vi "Analysis Dialog.vi"(8 "error in (no error)":errorcluster, 10 "Test Results":T5, 11 "Database in":refnum<queue>) -> (0 "error IO":errorcluster, 3 "Database out":refnum<queue>)   [LabVIEW 2026, in "Analysis.lvlib"]
uses:
  Analysis.lvlib
  Test Results.ctl
  Test Details.ctl
  support/Architecture/Message Queue/Message Cluster.ctl
  Hysteresis Result.ctl
  Repeatability Result.ctl
  Accuracy Result.ctl
  Linearity Result.ctl
  controls/UI/Analytics Refs.ctl
  controls/UI/UI List Type.ctl
  <vilib>/Utility/NIReport.llb/Report Type.ctl
  <vilib>/Utility/NIReport.llb/Append Text Table to Report (wrap).vi
  <vilib>/printing/OpenHTMLReport.llb/Open HTML Report in Browser (Refnum).vi
  <vilib>/Utility/NIReport.llb/NI_report.lvclass
  Settings/Settings.lvlib
  <vilib>/Utility/NIReport.llb/NI_ReportGenerationCore.lvlib
  support/Architecture/Message Queue/Message Queue.lvlib
panel:
  out "Temporary HTML file created":path
  in  "Generate Report":bool
  out "Max Deviations":dbl[](array[numeric])
  out "Linearity Results":T1[](array[typedef])
  out "Accuracy Results":T2[](array[typedef])
  out "Maximum Absolute Error":dbl
  out "Max Repeatability":dbl
  out "Repeatability Results":T3[](array[typedef])
  out "Max Hysteresis":dbl
  out "Hysteresis Results":T4[](array[typedef])
  in  "Exit":bool
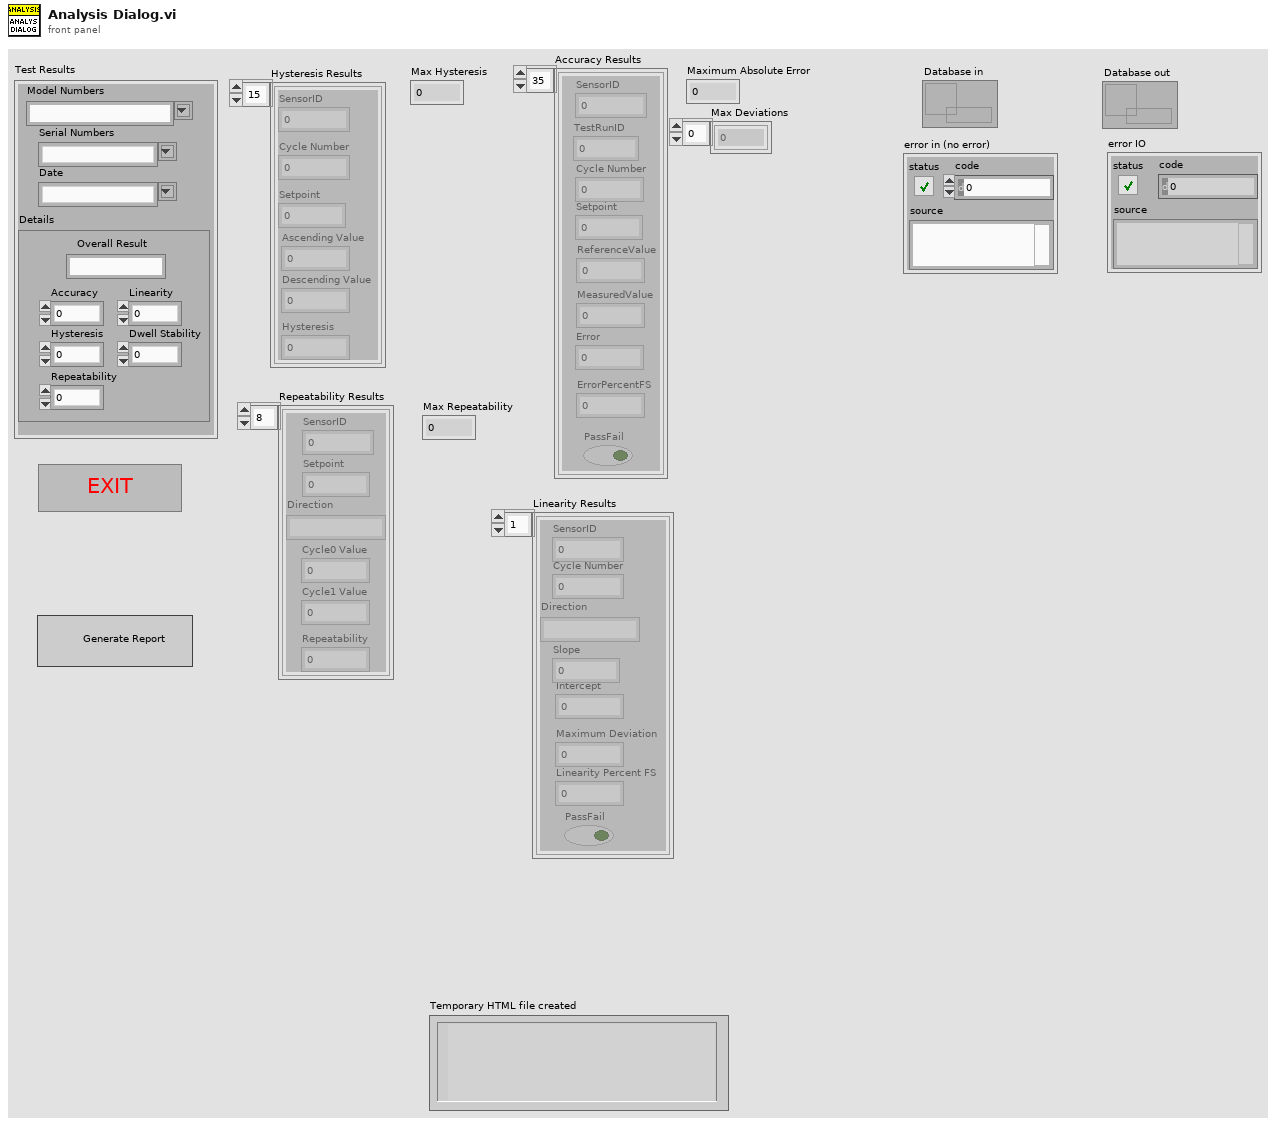
[diagram p1: front panel]
types:
  T1 = typedef "Analysis.lvlib/Linearity Result.ctl" = cluster{"Slope":dbl, "Intercept":dbl, "Cycle Number":i32, "SensorID":i32, "Maximum Deviation":dbl, "Linearity Percent FS":dbl, "Direction":string, "PassFail":bool}
  T2 = typedef "Analysis.lvlib/Accuracy Result.ctl" = cluster{"Setpoint":dbl, "Cycle Number":i32, "SensorID":i32, "TestRunID":i32, "ReferenceValue":dbl, "MeasuredValue":dbl, "ErrorPercentFS":dbl, "PassFail":bool, "Error":dbl}
  T3 = typedef "Analysis.lvlib/Repeatability Result.ctl" = cluster{"Setpoint":dbl, "Cycle0 Value":dbl, "SensorID":i32, "Cycle1 Value":dbl, "Repeatability":dbl, "Direction":string}
  T4 = typedef "Analysis.lvlib/Hysteresis Result.ctl" = cluster{"Setpoint":dbl, "Ascending Value":dbl, "Cycle Number":i32, "SensorID":i32, "Descending Value":dbl, "Hysteresis":dbl}
  T5 = typedef "Analysis.lvlib/Test Results.ctl" = cluster{"Model Numbers":string, "Serial Numbers":string, "Date":string, "Details":T6}
  T6 = typedef "Analysis.lvlib/Test Details.ctl" = cluster{"Accuracy":dbl, "Hysteresis":dbl, "Repeatability":dbl, "Linearity":dbl, "Dwell Stability":dbl, "Overall Result":string}
  T7 = typedef "Analysis.lvlib/Analytics Refs.ctl" = cluster{"Model Numbers Ref":refnum<vi>, "Serial Numbers Ref":refnum<vi>, "Date Ref":refnum<vi>, "Generate Report Ref":refnum<vi>}
  T8 = enum8{"Enabled", "Disabled", "Disabled and Grayed Out"}
  T9 = typedef "UI List Type.ctl" = enum16{"Model Numbers", "Serial Numbers", "Operators", "Calibration Points", "Start Run Times"}
  T10 = typedef "NI_ReportGenerationCore.lvlib/Report Type.ctl" = enum16{"HTML", "Word", "Excel"}
  T11 = typedef "Calibration Point Table Insert.ctl" = cluster{"TestRunID":i32, "ChannelRecordID":i32, "Setpoint":dbl, "MeasuredValue":dbl, "ErrorPercent":dbl, "PassFail":bool, "ReferenceValue":dbl, "Cycle Number":i32, "Direction":string, "SensorID":i32}
  T12 = typedef "Settings.lvlib/Sensor CoreData Cluster.ctl" = cluster{"SensorID":i32, "SerialNumber":string, "ModelNumber":string, "Min":dbl, "Max":dbl, "Units":T13, "Output Signal":T14}
  T13 = typedef "Units Enum.ctl" = enum16{"PSI", "Deg C", "kPa", "GPM"}
  T14 = typedef "Signal Enum.ctl" = enum16{"4-20mA", "0-10V", "Thermocouple Type K"}
  T15 = typedef "Analysis.lvlib/Full Scale Sensor Cluster.ctl" = cluster{"SensorID":i32, "FS":dbl}
  T16 = cluster{"Direction":string, "Cycle Number":i32, "SensorID":i32}[]
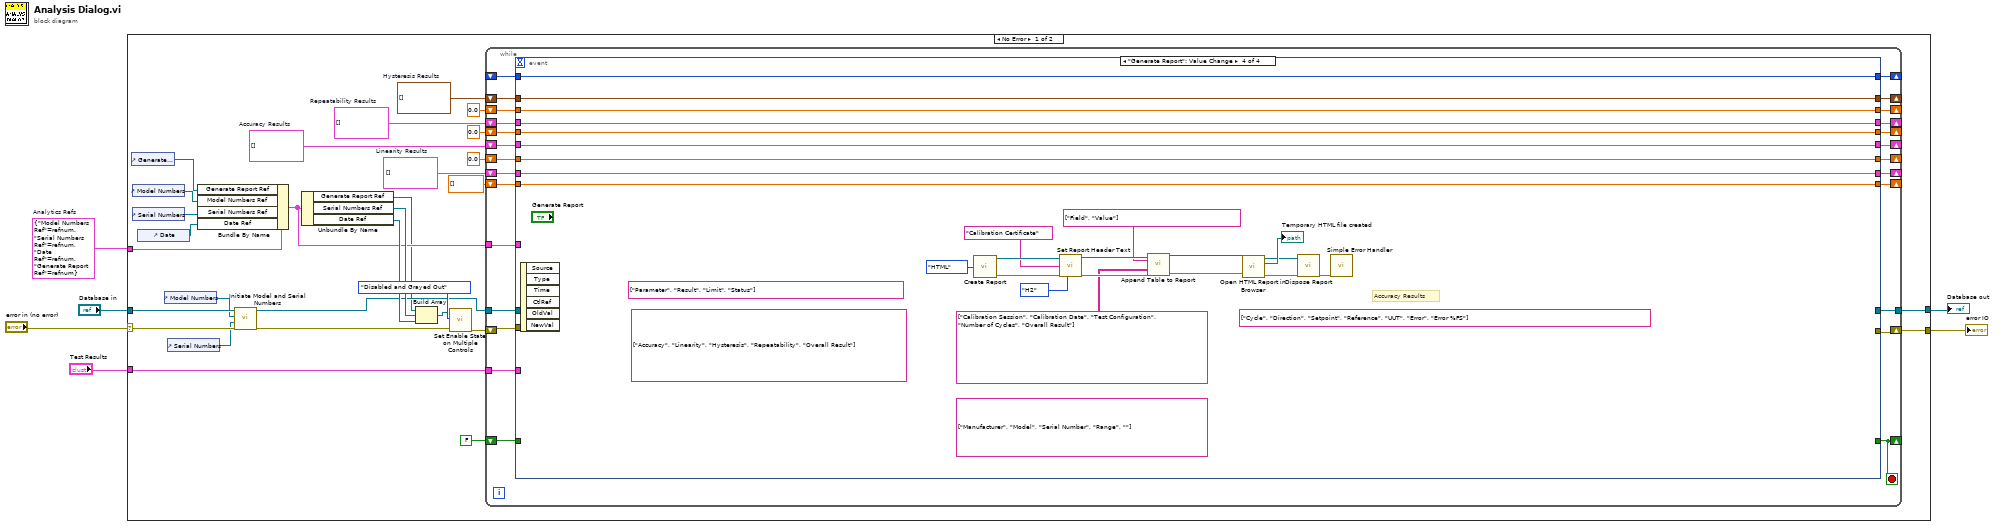
[diagram p0: block diagram]
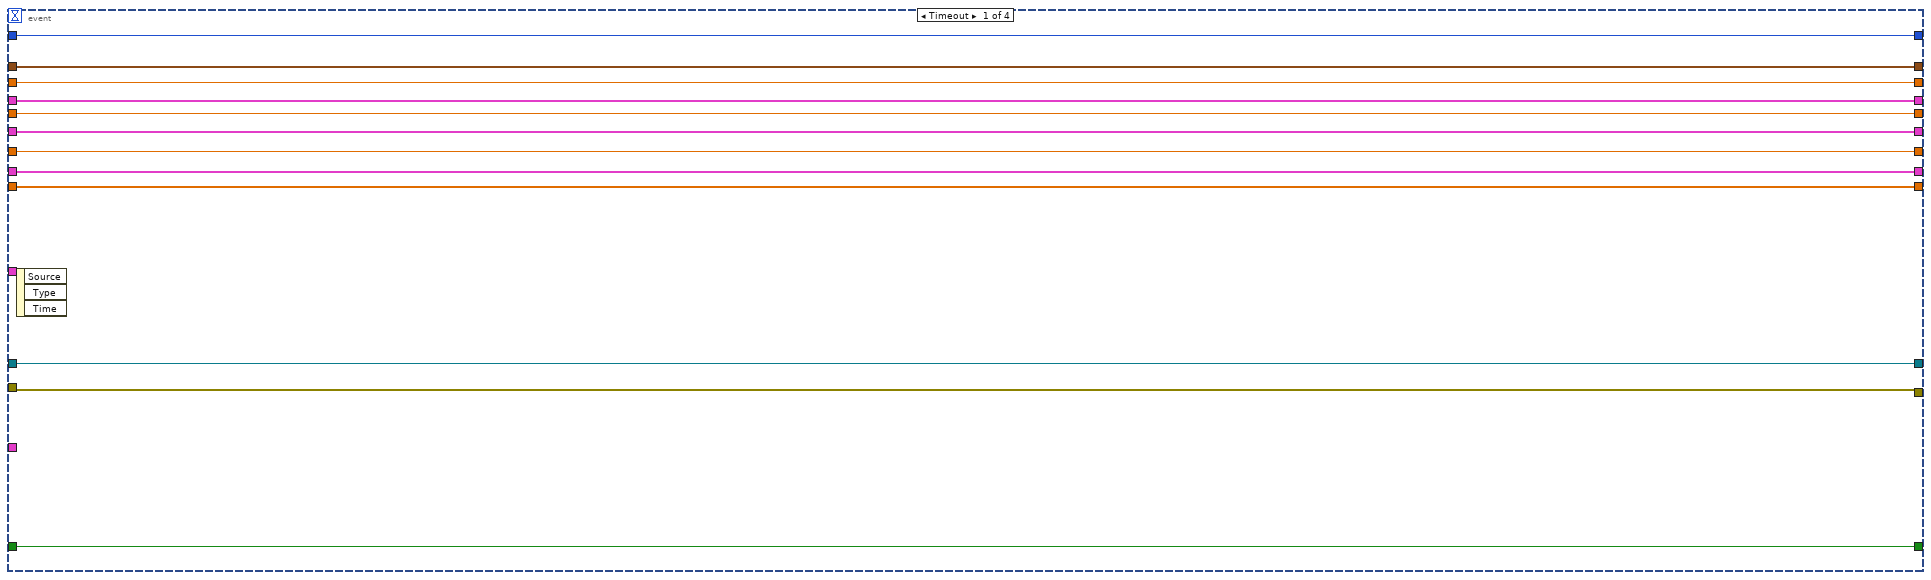
[diagram p2: hidden frame]
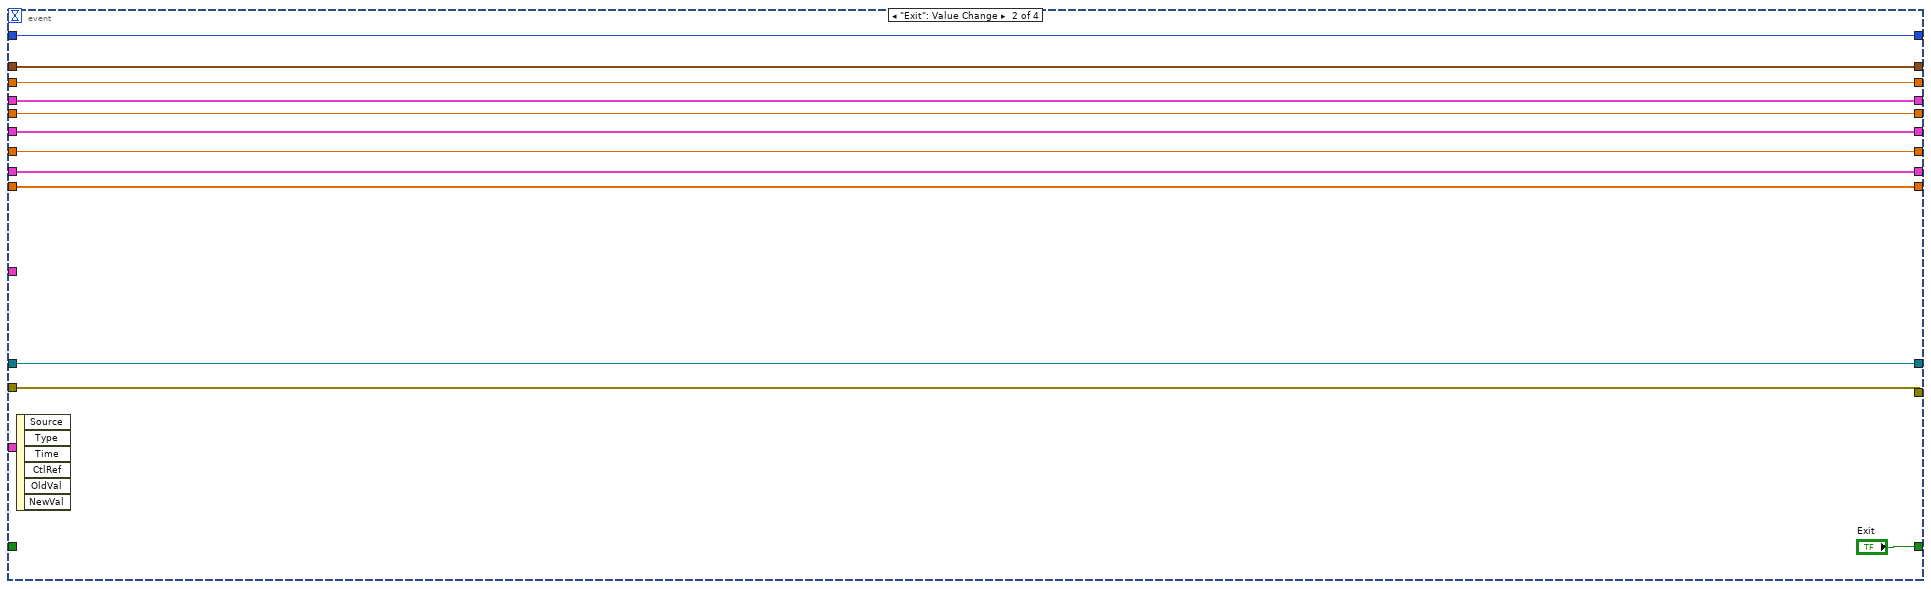
[diagram p3: hidden frame]
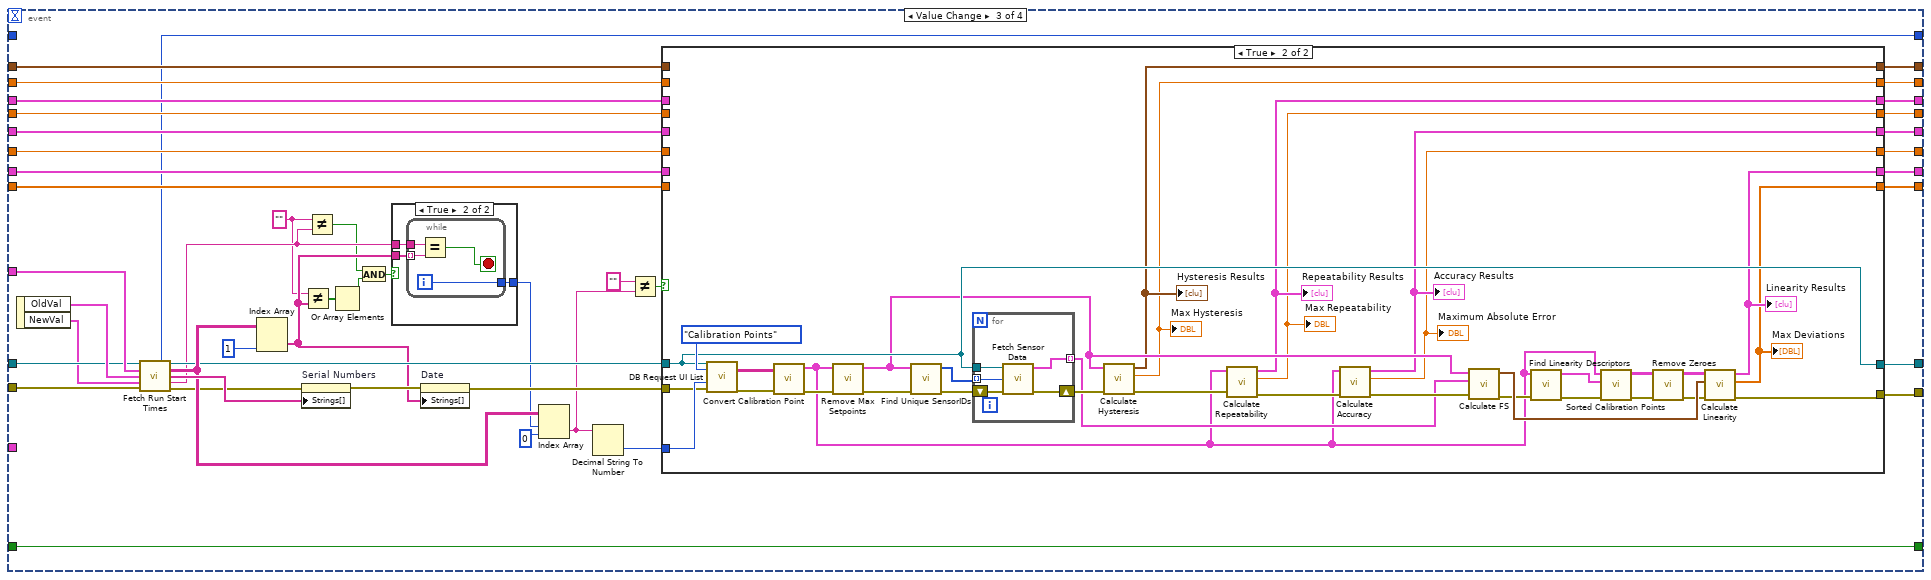
[diagram p4: hidden frame]
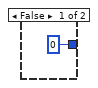
[diagram p5: hidden frame]
diagram:
  w1 = T7 {"Model Numbers Ref"=refnum, "Serial Numbers Ref"=refnum, "Date Ref"=refnum, "Generate Report Ref"=refnum}  # Analytics Refs
  n1 = case shown="No Error" "error in (no error)" {
    selector: "error in (no error)" -> [w32 w214]
    tunnel: [w35 w214] -> w5
    tunnel: "Database in" -> [w33 w213]
    tunnel: [w34 w213] -> w3
    tunnel: "Test Results" -> [w7 _]
    tunnel: w1 -> [w29 _]
    frame No Error {
      w11 = T1[] []  # Linearity Results
      w12 = T2[] []  # Accuracy Results
      w13 = T3[] []  # Repeatability Results
      w15 = T4[] []  # Hysteresis Results
      n2 = control-ref of="Generate Report"() -> (w17:refnum<vi>)
      n3 = control-ref of="Model Numbers"() -> (w28:refnum<vi>)
      n4 = control-ref of="Serial Numbers"() -> (w27:refnum<vi>)
      n5 = control-ref of="Date"() -> (w26:refnum<vi>)
      n6 = control-ref of="Model Numbers"() -> (w31:refnum<vi>)
      n7 = control-ref of="Serial Numbers"() -> (w30:refnum<vi>)
      n8 = Bundle By Name(cluster=w29, "Generate Report Ref"=w17, "Model Numbers Ref"=w28, "Serial Numbers Ref"=w27, "Date Ref"=w26) -> (w20:T7)
      n9 = call "Initiate Model and Serial Numbers.vi"("error in (no error)"=w32, "Serial CmbBox Ref"=w30, "Model CmbBox Ref"=w31, "Database in"=w33) -> ("error out"=w18:errorcluster, "Database out"=w19:refnum<queue>)  [unwired: 6 in]
      n10 = Unbundle By Name(w20) -> ("Generate Report Ref"=w16:refnum<vi>, "Serial Numbers Ref"=w24:refnum<vi>, "Date Ref"=w23:refnum<vi>)
      n11 = Build Array(w16, w24, w23) -> (w22:refnum<vi>[])
      n12 = call "Set Enable State on Multiple Controls.vi"("Controls"=w22, "Disabled"=T8."Disabled and Grayed Out", "error in (no error)"=w18) -> ("error out"=w21:errorcluster)  [unwired: 7 in]
      n13 = while {
        shift-right: [w61] -> w35
        shift-left: w21 -> [w57]
        shift-right: [w60] -> _
        shift-left: FALSE -> [w59]
        tunnel: [w62] -> w34
        tunnel: w19 -> [w58]
        tunnel: w20 -> [w56]
        shift-right: [w55] -> _
        shift-left: w15 -> [w47]
        shift-right: [w54] -> _
        shift-left: 0.0 ("Max Hysteresis") -> [w40]
        shift-right: [w53] -> _
        shift-left: w13 -> [w46]
        shift-right: [w52] -> _
        shift-left: 0.0 ("Max Repeatability") -> [w45]
        shift-right: [w51] -> _
        shift-left: w12 -> [w44]
        shift-right: [w50] -> _
        shift-left: 0.0 ("Maximum Absolute Error") -> [w43]
        shift-right: [w49] -> _
        shift-left: w11 -> [w42]
        shift-right: [w48] -> _
        shift-left: dbl[] [] ("Max Deviations") -> [w41]
        shift-right: [w39] -> _
        shift-left: _ -> [w38]
        tunnel: w7 -> [w37]
        stop <- w60 stop-if-true
        n14 = event shown="[3] \"Generate Report\": Value Change" {
          selector: _ -> [_ _ _ _]
          dyn-events: _ -> [_ _ _ _]
          timeout: _ -> [_ _ _ _]
          tunnel: w58 -> [w74 w86 w105 _]
          tunnel: w57 -> [w73 w85 w106 _]
          tunnel: [w74 w86 w123 _] -> w62
          tunnel: [w73 w85 w124 _] -> w61
          tunnel: [w72 "Exit" w130 _] -> w60
          tunnel: w59 -> [w72 _ w130 _]
          tunnel: w56 -> [_ _ w107 _]
          tunnel: [w71 w83 w103 w197] -> w55
          tunnel: [w70 w82 w102 w196] -> w54
          tunnel: [w69 w81 w101 w195] -> w53
          tunnel: [w68 w80 w100 w194] -> w52
          tunnel: [w67 w79 w99 w193] -> w51
          tunnel: [w66 w78 w98 w192] -> w50
          tunnel: [w65 w77 w97 w191] -> w49
          tunnel: [w64 w76 w96 w190] -> w48
          tunnel: w47 -> [w71 w83 w95 w197]
          tunnel: w46 -> [w69 w81 w94 w195]
          tunnel: w45 -> [w68 w80 w93 w194]
          tunnel: w44 -> [w67 w79 w91 w193]
          tunnel: w43 -> [w66 w78 w90 w192]
          tunnel: w42 -> [w65 w77 w89 w191]
          tunnel: w41 -> [w64 w76 w88 w190]
          tunnel: w40 -> [w70 w82 w92 w196]
          tunnel: [w63 w75 w87 w189] -> w39
          tunnel: w38 -> [w63 w75 _ w189]
          tunnel: w37 -> [_ _ _ _]
          event Timeout {
            n15 = event-data() -> ()  [unwired: 1 in, 3 out]
          }
          event "Exit": Value Change {
            n16 = event-data() -> ()  [unwired: 1 in, 6 out]
          }
          event Value Change {
            w113 = "" ("x")
            n17 = event-data() -> ("OldVal"=w108:T5, "NewVal"=w104:T5)  [unwired: 1 in]
            n18 = call "Fetch Run Start Times.vi"("Queue in"=w105, "Analytics Refs"=w107, "Old Value"=w108, "New Value"=w104, "error in (no error)"=w106) -> ("SensorID"=w87:i32, "Queue out"=w125:refnum<queue>, "Start Run Times"=w127:string[][], "Serial Numbers"=w131:string[], "Date"=w115:string, "error out"=w122:errorcluster)  [unwired: 4 in, 1 out]
            n19 = Index Array(array=w127, index (col)=1 ("index (row)")) -> (element=w114:string[])  [unwired: 1 in]
            n20 = property on="Serial Numbers" class="CmbBox"(error in=w122, "Strings[]"=w131) -> (error out=w121:errorcluster)  [unwired: 1 in, 1 out]
            n21 = Not Equal?(x=w113, y=w114) -> (x != y?=w111:bool[])
            n22 = Not Equal?(x=w113, y=w115) -> (x != y?=w112:bool)
            n23 = Or Array Elements(Boolean array=w111) -> (logical OR=w110:bool)
            n24 = And(x=w112, y=w110) -> (x .and. y?=w109:bool)
            n25 = case shown="True" w109 {
              tunnel: w114 -> [_ w135]
              tunnel: w115 -> [_ w134]
              tunnel: [0 w133] -> w116
              frame False {
              }
              frame True {
                n26 = while {
                  tunnel: w135 -> [w138] mode=indexing
                  tunnel: w134 -> [w139]
                  tunnel: [w136] -> w133
                  i -> [w136]
                  stop <- w137 stop-if-true
                  n27 = Equal?(x=w139, y=w138) -> (x = y?=w137:bool)
                }
              }
            }
            n28 = property on="Date" class="CmbBox"(error in=w121, "Strings[]"=w114) -> (error out=w120:errorcluster)  [unwired: 1 in, 1 out]
            n29 = Index Array(array=w127, index (row)=w116, index (col)=0 ("index (row)")) -> (element=w119:string)
            n30 = Decimal String To Number(string=w119) -> (number=w126:i32)  [unwired: 2 in, 1 out]
            n31 = Not Equal?(x="", y=w119) -> (x != y?=w117:bool)
            n32 = case shown="True" w117 {
              tunnel: w126 -> [_ w183]
              tunnel: w125 -> [w149 w172]
              tunnel: [w148 w171] -> w124
              tunnel: [w149 w172] -> w123
              tunnel: w120 -> [w148 w181]
              tunnel: [w147 w158] -> w103
              tunnel: [w146 w157] -> w102
              tunnel: [w145 w156] -> w101
              tunnel: [w144 w155] -> w100
              tunnel: [w143 w154] -> w99
              tunnel: [w142 w153] -> w98
              tunnel: [w141 w152] -> w97
              tunnel: [w140 w151] -> w96
              tunnel: w95 -> [w147 _]
              tunnel: w94 -> [w145 _]
              tunnel: w93 -> [w144 _]
              tunnel: w92 -> [w146 _]
              tunnel: w91 -> [w143 _]
              tunnel: w90 -> [w142 _]
              tunnel: w89 -> [w141 _]
              tunnel: w88 -> [w140 _]
              frame False {
              }
              frame True {
                n33 = call "DB Request UI List.vi"("Database in"=w172, "UI List Type"=UI_List_Type."Calibration Points", "Identifier"=w183, "error in (no error)"=w181) -> ("Results"=w180:string[][], "error out"=w179:errorcluster)  [unwired: 13 in, 1 out]
                n34 = call "Convert Calibration Point.vi"("error in (no error)"=w179, "DB Results"=w180) -> ("error out"=w178:errorcluster, "Conversion"=w150:T11[])  [unwired: 8 in]
                n35 = call "Remove Max Setpoints.vi"("error in (no error)"=w178, "Calibration Points in"=w150) -> ("error out"=w174:errorcluster, "Calibration Points out"=w168:T11[])  [unwired: 8 in]
                n36 = call "Find Unique SensorIDs.vi"("error in (no error)"=w174, "Calibration Points in"=w168) -> ("error out"=w173:errorcluster, "SensorIDs"=w175:i32[])  [unwired: 8 in]
                n37 = for {
                  tunnel: [w188] -> w167 mode=indexing
                  tunnel: w175 -> [w187] mode=indexing
                  tunnel: w172 -> [w186]
                  shift-right: [w184] -> w170
                  shift-left: w173 -> [w185]
                  n38 = call "Fetch Sensor Data.vi"("error in (no error)"=w185, "SensorID"=w187, "Database"=w186) -> ("error out"=w184:errorcluster, "Sensor CoreData Cluster"=w188:T12)  [unwired: 6 in, 1 out]
                }
                n39 = call "Calculate Hysteresis.vi"("error in (no error)"=w170, "Calibration Points"=w168) -> ("error out"=w177:errorcluster, "Max Hysteresis"=w157:dbl, "Hysteresis Results"=w158:T4[])  [unwired: 7 in]
                "Hysteresis Results" <- w158
                "Max Hysteresis" <- w157
                n40 = call "Calculate Repeatability.vi"("error in (no error)"=w177, "Calibration Points"=w150) -> ("error out"=w176:errorcluster, "Max Repeatability"=w155:dbl, "Repeatability Results"=w156:T3[])  [unwired: 7 in]
                "Repeatability Results" <- w156
                "Max Repeatability" <- w155
                n41 = call "Calculate Accuracy.vi"("error in (no error)"=w176, "Calibration Points"=w150) -> ("error out"=w169:errorcluster, "Maximum Absolute Error"=w153:dbl, "Accuracy Results"=w154:T2[])  [unwired: 7 in]
                "Maximum Absolute Error" <- w153
                "Accuracy Results" <- w154
                n42 = call "Calculate FS.vi"("error in (no error)"=w169, "Sensor CoreData"=w167, "Calibration Points"=w168) -> ("error out"=w164:errorcluster, "FS Sensors"=w166:T15[])  [unwired: 6 in]
                n43 = call "Find Linearity Descriptors.vi"("error in (no error)"=w164, "Calibration Points"=w150) -> ("error out"=w163:errorcluster, "Linearity Fit Descriptors"=w165:T16)  [unwired: 8 in]
                n44 = call "Sorted Calibration Points.vi"("error in (no error)"=w163, "Linearity Descriptors"=w165, "Calibration Points"=w150) -> ("error out"=w160:errorcluster, "Sorted Calibration Points"=w162:T11[][])  [unwired: 7 in]
                n45 = call "Remove Zeroes.vi"("error in (no error)"=w160, "Sorted Calibration Points"=w162) -> ("error out"=w159:errorcluster, "Zeroed Out Calibration Points"=w161:T11[][])  [unwired: 8 in]
                n46 = call "Calculate Linearity.vi"("error in (no error)"=w159, "FS Sensors"=w166, "Sorted Calibration Points"=w161) -> ("error out"=w171:errorcluster, "Max Deviations"=w151:dbl[], "Linearity Results"=w152:T1[])  [unwired: 6 in]
                "Linearity Results" <- w152
                "Max Deviations" <- w151
              }
            }
          }
          event "Generate Report": Value Change {
            (unwired) string[] ["Cycle", "Direction", "Setpoint", "Reference", "UUT", "Error", "Error %FS"] ("column headers")
            (unwired) string[] ["Parameter", "Result", "Limit", "Status"] ("column headers")
            (unwired) string[][] [["Accuracy"], ["Linearity"], ["Hysteresis"], ["Repeatability"], ["Overall Result"]] ("Array")
            (unwired) string[][] [["Manufacturer"], ["Model"], ["Serial Number"], ["Range"], [""]] ("Array")
            # "Accuracy Results"
            n47 = event-data() -> ()  [unwired: 1 in, 6 out]
            n48 = call <vilib>:"Create Report.vi"("report type"=Report_Type."HTML") -> ("report out"=w208:refnum<class "NI_report.lvclass">, "error out"=w207:errorcluster)  [unwired: 13 in]
            n49 = call-dynamic "Set Report Header Text.vi"("report in"=w208, "center header text"="Calibration Certificate", "error in (no error)"=w207, "HTML header size"=enum16{"H1", "H2", "H3", "H4", "H5", "H6", "H7"}."H2") -> ("report out"=w211:refnum<class "NI_report.lvclass">, "error out"=w209:errorcluster)  [unwired: 10 in]
            n50 = call-poly <vilib>:"Append Table to Report.vi"("report in"=w211, "column headers"=string[] ["Field", "Value"], "text data"=string[][] [["Calibration Session"], ["Calibration Date"], ["Test Configuration"], ["Number of Cycles"], ["Overall Result"]] ("Array"), "error in (no error)"=w209) -> ("report out"=w212:refnum<class "NI_report.lvclass">, "error out"=w210:errorcluster)  [unwired: 8 in, 2 out]
            n51 = call-poly <vilib>:"Open HTML Report in Browser.vi"("report in"=w212, "error in (no error)"=w210) -> ("report out"=w204:refnum<class "NI_report.lvclass">, "temporary HTML file created"=→"Temporary HTML file created":path, "error out"=w203:errorcluster)  [unwired: 11 in]
            n52 = call-dynamic "Dispose Report.vi"("report in"=w204, "error in (no error)"=w203) -> ("error out"=w202:errorcluster)  [unwired: 13 in]
            n53 = call <vilib>:"Simple Error Handler.vi"("error in (no error)"=w202) -> ()  [unwired: 4 in, 5 out]
          }
        }
      }
    }
    frame Error {
    }
  }
  "error IO" <- w5
  "Database out" <- w3
